vi "Set Float.vi"(8 "error in (no error)":errorcluster, 10 "Float Mode":T1, 11 "SR7270 Drivers in":refnum<class "SR7270 Drivers.lvclass">) -> (0 "error out":errorcluster, 3 "SR7270 Drivers out":refnum<class "SR7270 Drivers.lvclass">)   [LabVIEW 2016, in "SR7270 Drivers.lvclass"]
uses:
  SR7270 Drivers.lvclass
  Typedefs/FLOAT--enum.ctl
  SR7270 Drivers.lvclass/SR7270 Drivers.ctl
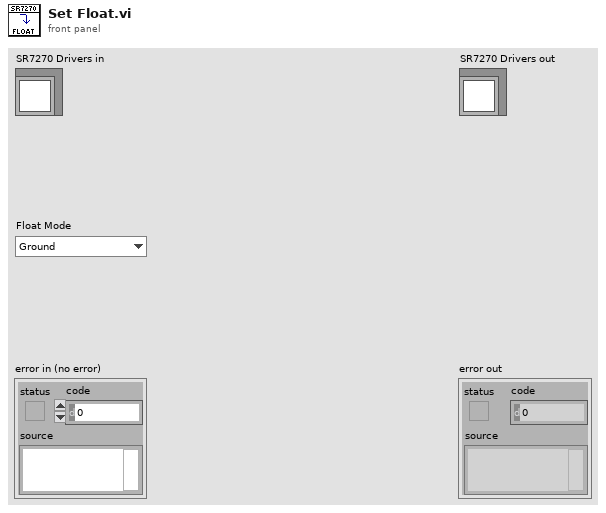
[diagram p1: front panel]
types:
  T1 = typedef "SR7270 Drivers.lvclass/FLOAT--enum.ctl" = enum16{"Ground", "Float"}
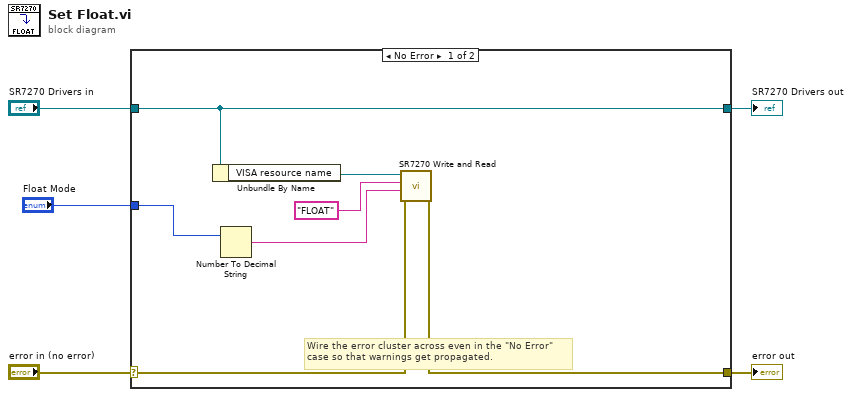
[diagram p0: block diagram]
diagram:
  n1 = case shown="No Error" "error in (no error)" {
    selector: "error in (no error)" -> [w10 w14]
    tunnel: [w9 w14] -> w4
    tunnel: [w11 w13] -> w2
    tunnel: "SR7270 Drivers in" -> [w11 w13]
    tunnel: "Float Mode" -> [w7 _]
    frame No Error {
      # "Wire the error cluster across even in the \"No Error\"\ncase so that warnings get propagated."
      n2 = Unbundle By Name(w11) -> ("VISA resource name"=w12:refnum<visa-resource-name>)
      n3 = Number To Decimal String(number=w7) -> (decimal integer string=w6:string)  [unwired: 1 in]
      n4 = call "SR7270 Write and Read.vi"("error in (no error)"=w10, "Parameter(s)"=w6, "Command Name"="FLOAT", "VISA resource name"=w12) -> ("error out"=w9:errorcluster)  [unwired: 4 in, 3 out]
    }
    frame Error {
    }
  }
  "error out" <- w4
  "SR7270 Drivers out" <- w2
